vi "בדיקת מתח תפיסה של סליל פיקוד ללא עומס 5.vi"(8 "error":errorcluster, 10 "lines":tag="PXI1Slot8/port0/line1", 11 "Path for Log":path) -> (0 "error out":errorcluster, 1 "מצב ממסר פתוח/סגור":bool, 2 "מתח סגירת הממסר":dbl format="%.4f", 3 "מתח מוצא מהספק":dbl format="%.4f", 5 "resultUserPrompt":bool)   [LabVIEW 2014]
uses:
  <vilib>/DAQmx/create/channels.llb/DAQmx Create Channel (DO-Digital Output).vi
  <vilib>/DAQmx/write.llb/DAQmx Write (Digital Bool 1Line 1Point).vi
panel:
  out "progress":dbl(slide) scale=0.0..36.0
  out "error IO DMM":errorcluster
  in  "Stop Button":bool
  # "Right-Click to\nexplain error"
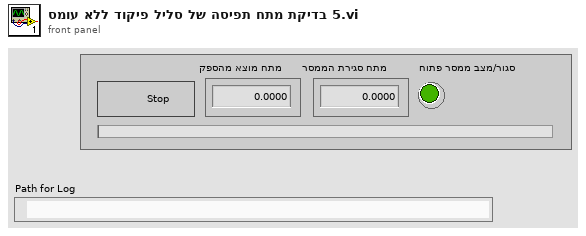
[diagram p1: front panel]
types:
  T1 = enum32{"Invalid", "Standard", "Closed", "Hidden", "Minimized", "Maximized"}
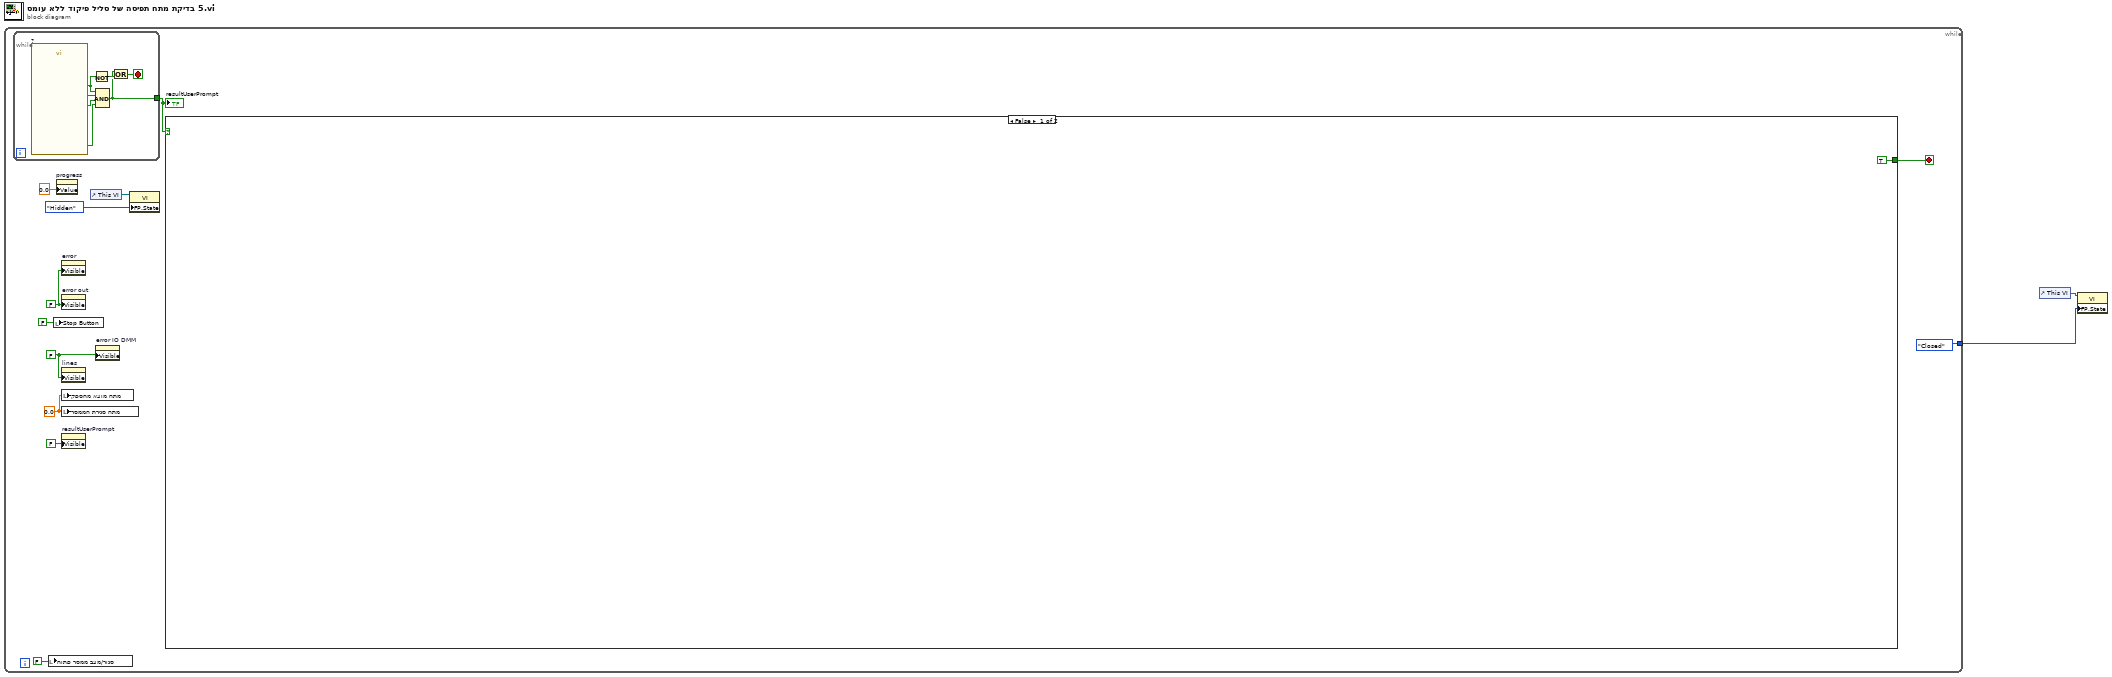
[diagram p0: block diagram]
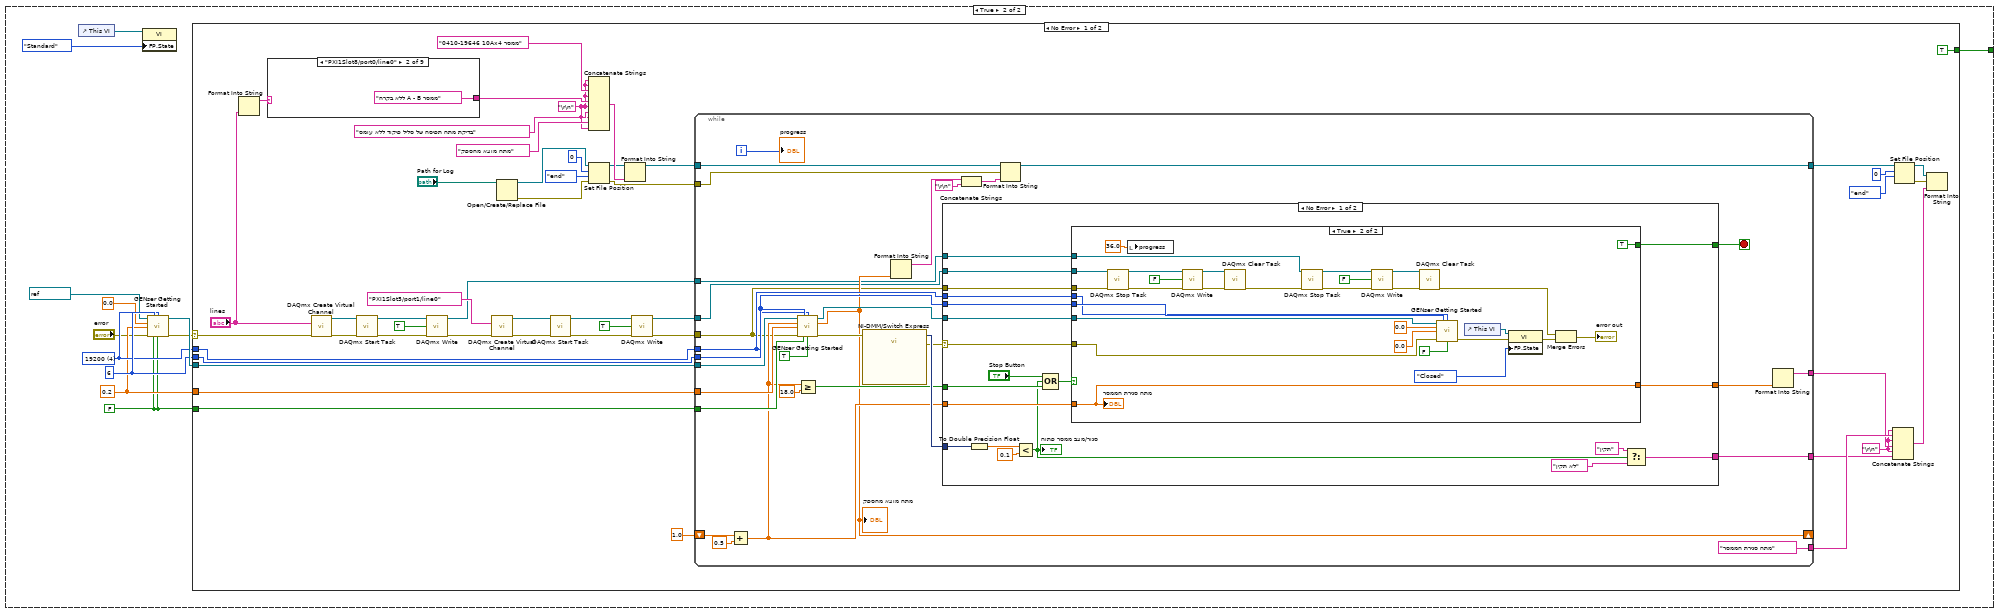
[diagram p2: hidden frame]
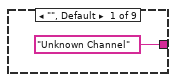
[diagram p3: hidden frame]
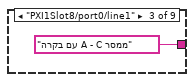
[diagram p4: hidden frame]
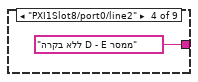
[diagram p5: hidden frame]
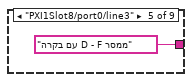
[diagram p6: hidden frame]
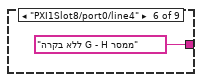
[diagram p7: hidden frame]
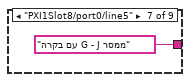
[diagram p8: hidden frame]
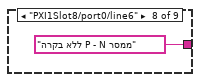
[diagram p9: hidden frame]
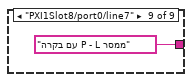
[diagram p10: hidden frame]
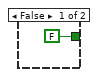
[diagram p11: hidden frame]
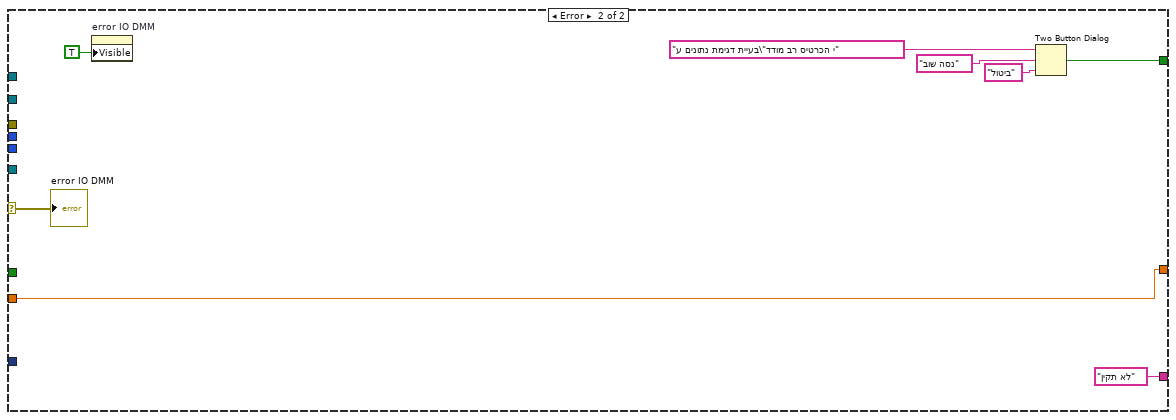
[diagram p12: hidden frame]
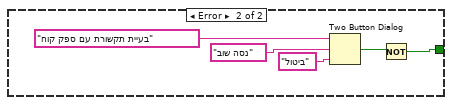
[diagram p13: hidden frame]
diagram:
  n1 = while {
    tunnel: [T1."Closed" ("Front Panel Window:State")] -> w1
    stop <- w4 stop-if-true
    w7 = FALSE ("Visible")
    w10 = 0.0 ("signals out")
    w5 = FALSE ("Visible")
    n2 = while {
      tunnel: [w15] -> w14
      stop <- w16 stop-if-true
      n3 = call "?"() -> ("הדקי הרב מודד"=w19:bool, "M מגע שלילי"=w20:bool, "K מגע חיובי"=w21:bool, "OK"=w17:bool)  [unwired: 15 in, 1 out]
      n4 = Not(x=w17) -> (.not. x?=w18:bool)
      n5 = Compound Arithmetic op=AND(w17, w21, w20, w19) -> (w15:bool)
      n6 = Or(x=w15, y=w18) -> (x .or. y?=w16:bool)
    }
    "resultUserPrompt" <- w14
    n7 = local write "מצב ממסר פתוח/סגור"(FALSE ("מגע סגור")) -> ()
    n8 = local write "Stop Button"(FALSE ("Reset (T)")) -> ()
    n9 = property on="progress" class="Slide (strict)"("Value"=0.0 ("progress")) -> ()  [unwired: 2 in, 2 out]
    n10 = property on="error" class="Clust (strict)"("Visible"=w7) -> ()  [unwired: 2 in, 2 out]
    n11 = property on="error out" class="Clust (strict)"("Visible"=w7) -> ()  [unwired: 2 in, 2 out]
    n12 = property on="lines" class="DAQmxName"("Visible"=w5) -> ()  [unwired: 2 in, 2 out]
    n13 = local write "מתח מוצא מהספק"(w10) -> ()
    n14 = local write "מתח סגירת הממסר"(w10) -> ()
    n15 = property on="resultUserPrompt" class="Bool (strict)"("Visible"=FALSE) -> ()  [unwired: 2 in, 2 out]
    n16 = control-ref of="This VI"() -> (w9:refnum<vi>)
    n17 = property on="error IO DMM" class="Clust (strict)"("Visible"=w5) -> ()  [unwired: 2 in, 2 out]
    n18 = property class="VI"(reference=w9, "FP.State"=T1."Hidden" ("Front Panel Window:State")) -> ()  [unwired: 1 in, 2 out]
    n19 = case shown="False" w14 {
      tunnel: [TRUE ("T button?") w28] -> w4
      frame False {
      }
      frame True {
        w27 = FALSE ("Output On (T)")
        w32 = u16 4 items=["1200", "2400", "4800", "9600", "19200"] ("BAUD")
        w33 = i16 6 ("GEN Addr")
        w29 = 0.2 ("Current Limit")
        n20 = control-ref of="This VI"() -> (w25:refnum<vi>)
        n21 = property class="VI"(reference=w25, "FP.State"=T1."Standard" ("Front Panel Window:State")) -> ()  [unwired: 1 in, 2 out]
        n22 = call "GENser Getting Started.vi"("VISA"=refnum<visa-resource-name> "COM6", "GEN Addr"=w33, "BAUD"=w32, "Voltage Limit"=0.0, "Current Limit"=w29, "error"="error", "Reset (T)"=w27, "Output On (T)"=w27) -> ("VISA out"=w34:refnum<visa-resource-name>, "error out"=w24:errorcluster)  [unwired: 4 in, 2 out]
        n23 = case shown="No Error" w24 {
          selector: w24 -> [w51 _]
          tunnel: w34 -> [w83 _]
          tunnel: w33 -> [w82 _]
          tunnel: w32 -> [w81 _]
          tunnel: w27 -> [w80 _]
          tunnel: w29 -> [w79 _]
          tunnel: [TRUE w183] -> w28
          frame No Error {
            w35 = "\r\n"
            w73 = "\r\n"
            n24 = Format Into String("lines") -> (resulting string=w39:string)  [unwired: 3 in, 1 out]
            n25 = case shown="\"PXI1Slot8/port0/line0\"" w39 {
              tunnel: ["Unknown Channel" "ללא בקרה A - B ממסר" "עם בקרה A - C ממסר" "ללא בקרה D - E ממסר" "עם בקרה D - F ממסר" "ללא בקרה G - H ממסר" "עם בקרה G - J ממסר" "ללא בקרה P - N ממסר" "עם בקרה P - L ממסר"] -> w37
              frame "", Default {
              }
              frame "PXI1Slot8/port0/line0" {
              }
              frame "PXI1Slot8/port0/line1" {
              }
              frame "PXI1Slot8/port0/line2" {
              }
              frame "PXI1Slot8/port0/line3" {
              }
              frame "PXI1Slot8/port0/line4" {
              }
              frame "PXI1Slot8/port0/line5" {
              }
              frame "PXI1Slot8/port0/line6" {
              }
              frame "PXI1Slot8/port0/line7" {
              }
            }
            n26 = call-poly <vilib>:"DAQmx Create Virtual Channel.vi"("lines"="lines", "error in"=w51) -> ("task out"=w56:refnum<k21>, "error out"=w55:errorcluster)  [unwired: 12 in]
            n27 = call <vilib>:"DAQmx Start Task.vi"("task/channels in"=w56, "error in"=w55) -> ("task out"=w53:refnum<k21>, "error out"=w54:errorcluster)  [unwired: 12 in]
            n28 = call-poly <vilib>:"DAQmx Write.vi"("task/channels in"=w53, "data"=TRUE, "error in"=w54) -> ("task out"=w40:refnum<k21>, "error out"=w50:errorcluster)  [unwired: 10 in, 1 out]
            n29 = call-poly <vilib>:"DAQmx Create Virtual Channel.vi"("lines"=tag "PXI1Slot5/port1/line0", "error in"=w50) -> ("task out"=w63:refnum<k21>, "error out"=w64:errorcluster)  [unwired: 12 in]
            n30 = Open/Create/Replace File(file path (use dialog)="Path for Log") -> (refnum out=w47:refnum<file>, error out=w46:errorcluster)  [unwired: 5 in, 1 out]
            n31 = call <vilib>:"DAQmx Start Task.vi"("task/channels in"=w63, "error in"=w64) -> ("task out"=w60:refnum<k21>, "error out"=w59:errorcluster)  [unwired: 12 in]
            n32 = Concatenate Strings(w35, w35, "0410-19646 10Ax4 ממסר", w35, w37, w35, "בדיקת מתח תפיסה של סליל פיקוד ללא עומס", w35, "מתח מוצא מהספק", w35) -> (w45:string)
            n33 = Set File Position(offset (in bytes) (0)=i64 0, refnum=w47, from (0:start)=enum16{"start", "end", "current"}."end", error in=w46) -> (refnum out=w42:refnum<file>, error out=w66:errorcluster)
            n34 = Format Into String(initial string=w42, w45) -> (resulting string=w65:refnum<file>)  [unwired: 2 in, 1 out]
            n35 = call-poly <vilib>:"DAQmx Write.vi"("task/channels in"=w60, "data"=TRUE, "error in"=w59) -> ("task out"=w58:refnum<k21>, "error out"=w57:errorcluster)  [unwired: 10 in, 1 out]
            n36 = while {
              tunnel: w83 -> [w113]
              tunnel: w82 -> [w115]
              tunnel: w81 -> [w114]
              tunnel: w80 -> [w123]
              tunnel: w79 -> [w121]
              shift-right: [w105] -> _
              shift-left: 1.0 ("y") -> [w119]
              tunnel: ["מתח סגירת הממסר"] -> w76
              tunnel: [w103] -> w75
              tunnel: [w102] -> w74
              tunnel: [w99] -> w72
              tunnel: w65 -> [w98]
              tunnel: w66 -> [w97]
              tunnel: w58 -> [w95]
              tunnel: w57 -> [w94]
              tunnel: w40 -> [w93]
              i -> [w106]
              stop <- w116 stop-if-true
              n37 = Add(x=w119, y=0.5) -> (x+y=w107:dbl)
              n38 = call "GENser Getting Started.vi"("VISA"=w113, "GEN Addr"=w115, "BAUD"=w114, "Voltage Limit"=w107, "Current Limit"=w121, "error"=w94, "Reset (T)"=w123, "Output On (T)"=TRUE) -> ("VISA out"=w112:refnum<visa-resource-name>, "Output Voltage"=w105:dbl, "error out"=w118:errorcluster)  [unwired: 4 in, 1 out]
              "מתח מוצא מהספק" <- w105
              n39 = Greater Or Equal?(x=w107, y=18.0) -> (x >= y?=w110:bool)
              n40 = call "NI-DMM/Switch Express"("error in"=w118) -> ("signals out"=w117:dynamicdata, "error out"=w109:errorcluster)  [unwired: 16 in, 1 out]
              n41 = Format Into String(w105) -> (resulting string=w100:string)  [unwired: 3 in, 1 out]
              n42 = case shown="No Error" w109 {
                selector: w109 -> [w135 w182]
                tunnel: w117 -> [w143 _]
                tunnel: [w132 w178] -> w116
                tunnel: w115 -> [w140 _]
                tunnel: w114 -> [w139 _]
                tunnel: w112 -> [w138 _]
                tunnel: w110 -> [w137 _]
                tunnel: w107 -> [w136 w176]
                tunnel: [w131 w176] -> w108
                tunnel: [w128 "לא תקין"] -> w102
                tunnel: w95 -> [w126 _]
                tunnel: w94 -> [w125 _]
                tunnel: w93 -> [w124 _]
                frame No Error {
                  n43 = To Double Precision Float(number=w143) -> (double precision float=w134:dbl)
                  n44 = Less?(x=w134, y=0.1) -> (x < y?=w127:bool)
                  "מצב ממסר פתוח/סגור" <- w127
                  n45 = Compound Arithmetic op=OR("Stop Button", w127, w137) -> (w142:bool)
                  n46 = case shown="True" w142 {
                    tunnel: [FALSE TRUE] -> w132
                    tunnel: w140 -> [_ w174]
                    tunnel: w139 -> [_ w173]
                    tunnel: w138 -> [_ w172]
                    tunnel: w135 -> [_ w169]
                    tunnel: w136 -> [_ w164]
                    tunnel: [_ w164] -> w131
                    tunnel: w126 -> [_ w155]
                    tunnel: w125 -> [_ w154]
                    tunnel: w124 -> [_ w145]
                    frame False {
                    }
                    frame True {
                      n47 = call <vilib>:"DAQmx Stop Task.vi"("task/channels in"=w155, "error in"=w154) -> ("task out"=w162:refnum<k21>, "error out"=w160:errorcluster)  [unwired: 12 in]
                      n48 = local write "progress"(36.0 ("progress")) -> ()
                      n49 = call-poly <vilib>:"DAQmx Write.vi"("task/channels in"=w162, "data"=FALSE, "error in"=w160) -> ("task out"=w159:refnum<k21>, "error out"=w158:errorcluster)  [unwired: 10 in, 1 out]
                      n50 = call <vilib>:"DAQmx Clear Task.vi"("task in"=w159, "error in"=w158) -> ("error out"=w147:errorcluster)  [unwired: 13 in]
                      n51 = call <vilib>:"DAQmx Stop Task.vi"("task/channels in"=w145, "error in"=w147) -> ("task out"=w148:refnum<k21>, "error out"=w150:errorcluster)  [unwired: 12 in]
                      n52 = call-poly <vilib>:"DAQmx Write.vi"("task/channels in"=w148, "data"=FALSE, "error in"=w150) -> ("task out"=w151:refnum<k21>, "error out"=w152:errorcluster)  [unwired: 10 in, 1 out]
                      n53 = call <vilib>:"DAQmx Clear Task.vi"("task in"=w151, "error in"=w152) -> ("error out"=w146:errorcluster)  [unwired: 13 in]
                      n54 = call "GENser Getting Started.vi"("VISA"=w172, "GEN Addr"=w174, "BAUD"=w173, "Voltage Limit"=0.0, "Current Limit"=0.0, "error"=w169, "Output On (T)"=FALSE) -> ("error out"=w153:errorcluster)  [unwired: 5 in, 3 out]
                      n55 = control-ref of="This VI"() -> (w166:refnum<vi>)
                      n56 = property class="VI"(reference=w166, error in=w153, "FP.State"=T1."Closed" ("Front Panel Window:State")) -> (error out=w156:errorcluster)  [unwired: 1 out]
                      n57 = Merge Errors(w146, w156) -> (→"error out":errorcluster)
                      "מתח סגירת הממסר" <- w164
                    }
                  }
                  n58 = Select(t="תקין", s=w127, f="לא תקין") -> (s? t:f=w128:string)
                }
                frame Error {
                  n59 = property on="error IO DMM" class="Clust (strict)"("Visible"=TRUE) -> ()  [unwired: 2 in, 2 out]
                  n60 = Two Button Dialog(message="בעיית דגימת נתונים ע\"י הכרטיס רב מודד", 1:"ביטול" ("F button name (\"Cancel\")"), 2:"נסה שוב" ("T button name (\"OK\")")) -> (T button?=w178:bool)
                  "error IO DMM" <- w182
                }
              }
              n61 = Concatenate Strings(w100, "\r\n") -> (w96:string)
              n62 = Format Into String(initial string=w98, error in=w97, w96) -> (resulting string=w99:refnum<file>)  [unwired: 1 in, 1 out]
              n63 = Format Into String(w108) -> (resulting string=w103:string)  [unwired: 3 in, 1 out]
              "progress" <- w106
            }
            n64 = Concatenate Strings(w73, w76, w73, w75, w73, w74) -> (w67:string)
            n65 = Set File Position(offset (in bytes) (0)=i64 0, refnum=w72, from (0:start)=enum16{"start", "end", "current"}."end") -> (refnum out=w69:refnum<file>, error out=w68:errorcluster)  [unwired: 1 in]
            n66 = Format Into String(initial string=w69, error in=w68, w67) -> ()  [unwired: 1 in, 2 out]
          }
          frame Error {
            n67 = Two Button Dialog(message="בעיית תקשורת עם ספק קוח", 1:"ביטול" ("F button name (\"Cancel\")"), 2:"נסה שוב" ("T button name (\"OK\")")) -> (T button?=w184:bool)
            n68 = Not(x=w184) -> (.not. x?=w183:bool)
          }
        }
      }
    }
  }
  n69 = control-ref of="This VI"() -> (w2:refnum<vi>)
  n70 = property class="VI"(reference=w2, "FP.State"=w1) -> ()  [unwired: 1 in, 2 out]
